vi "SRV_VIG_XModem Updates in Progress.vi"(7 "XModem Updates in Progress":bool, 11 "error in (no error)":errorcluster, 12 "Method (Get)":enum16{"Get", "Set"}(ring)) -> (8 "XModem Updates in Progress?":bool, 15 "error out":errorcluster)   [LabVIEW 2014]
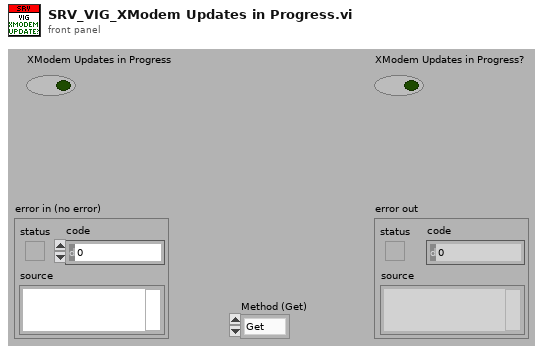
[diagram p1: front panel]
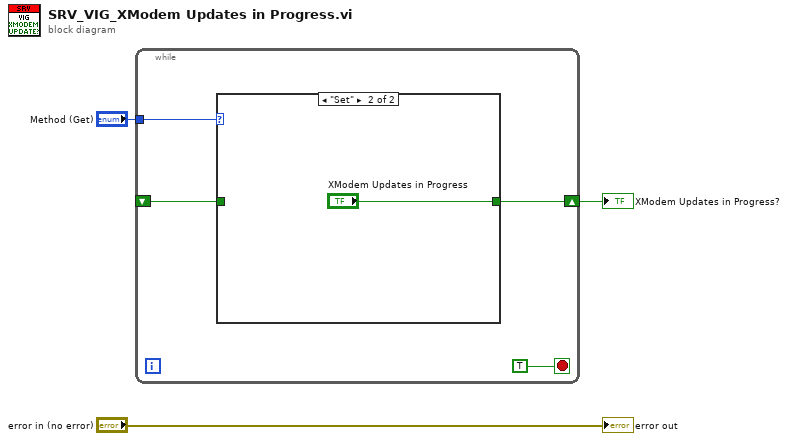
[diagram p0: block diagram]
diagram:
  n1 = while {
    tunnel: "Method (Get)" -> [w7]
    shift-right: [w5] -> w2
    shift-left: _ -> [w6]
    stop <- TRUE stop-if-true
    n2 = case shown="\"Set\"" w7 {
      tunnel: w6 -> [w8 _]
      tunnel: [w8 "XModem Updates in Progress"] -> w5
      frame "Get" {
      }
      frame "Set" {
      }
    }
  }
  "XModem Updates in Progress?" <- w2
  "error out" <- "error in (no error)"
